vi "loginOrRegister.vi"(8 "error in":errorcluster, 10 "passwd":string, 11 "uname":string) -> (0 "error out":errorcluster, 3 "OK?":bool)   [LabVIEW 2024]
uses:
  user_name.vi
  session.vi
  <vilib>/regexp/Match Regular Expression.xnode
  <vilib>/httpClient/LabVIEWHTTPClient.lvlib
panel:
  # "Login Or Register"
  # "Login or register to server, check internet status,\nafter successfully logged in, save session as global variable, save user name as global variable, download user avatar from server"
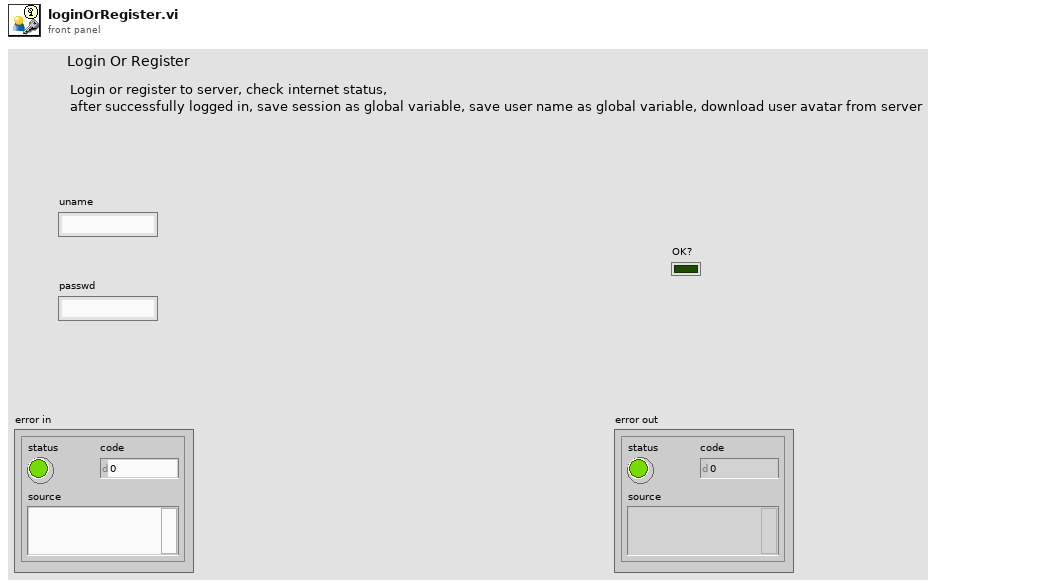
[diagram p1: front panel]
types:
  T1 = typedef "LabVIEWHTTPClient.lvlib/ClientHandle.ctl" = refnum<k1>
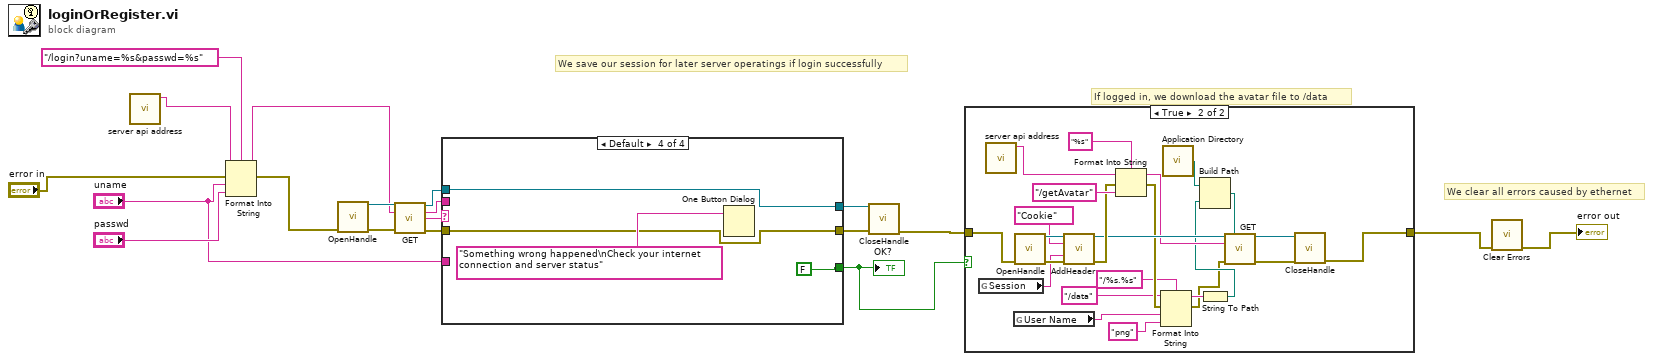
[diagram p0: block diagram]
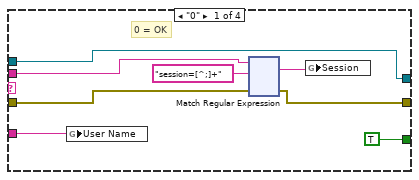
[diagram p2: hidden frame]
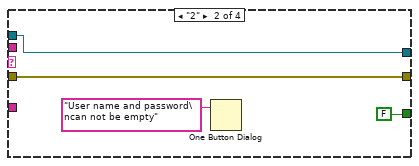
[diagram p3: hidden frame]
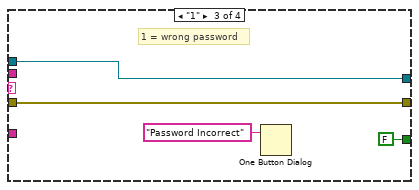
[diagram p4: hidden frame]
diagram:
  # "We clear all errors caused by ethernet"
  # "If logged in, we download the avatar file to /data"
  # "We save our session for later server operatings if login successfully"
  n1 = call "server api address.vi"() -> ("Server API URL"=w4:string)  [unwired: 11 in]
  n2 = Format Into String(format string="/login?uname=%s&passwd=%s", initial string=w4, error in="error in", "uname", "passwd") -> (resulting string=w17:string, error out=w14:errorcluster)
  n3 = call <vilib>:"OpenHandle.vi"("error in (no error)"=w14) -> ("client handle out"=w18:T1, "error out"=w19:errorcluster)  [unwired: 13 in]
  n4 = call <vilib>:"GET.vi"("client handle"=w18, "url"=w17, "error in (no error)"=w19) -> ("client handle out"=w11:T1, "headers"=w12:string, "body"=w13:string, "error out"=w10:errorcluster)  [unwired: 9 in]
  n5 = case shown="Default" w13 {
    tunnel: w12 -> [w24 _ _ _]
    tunnel: w11 -> [w21 w148 w151 w154]
    tunnel: w10 -> [w23 w147 w150 w155]
    tunnel: [TRUE FALSE FALSE FALSE] -> w6
    tunnel: [w21 w148 w151 w154] -> w9
    tunnel: [w22 w147 w150 w155] -> w8
    tunnel: "uname" -> [w20 _ _ _]
    frame "0" {
      # "0 = OK"
      n6 = global write "user_name.vi" "User Name"(w20) -> ()
      n7 = xnode "Match Regular Expression"("input string"=w24, "regular expression"="session=[^;]+", "error in"=w23) -> ("whole match"=w25:string, "error out"=w22:errorcluster)  [unwired: 3 in, 3 out]
      n8 = global write "session.vi" "Session"(w25) -> ()
    }
    frame "2" {
      n9 = One Button Dialog(message="User name and password\ncan not be empty") -> ()  [unwired: 1 in, 1 out]
    }
    frame "1" {
      # "1 = wrong password"
      n10 = One Button Dialog(message="Password Incorrect") -> ()  [unwired: 1 in, 1 out]
    }
    frame Default {
      n11 = One Button Dialog(message="Something wrong happened\nCheck your internet connection and server status") -> ()  [unwired: 1 in, 1 out]
    }
  }
  "OK?" <- w6
  n12 = call <vilib>:"CloseHandle.vi"("client handle"=w9, "error in (no error)"=w8) -> ("error out"=w3:errorcluster)  [unwired: 13 in]
  n13 = case shown="True" w6 {
    tunnel: w3 -> [w157 w181]
    tunnel: [w157 w170] -> w1
    frame False {
    }
    frame True {
      n14 = global read "session.vi" "Session"() -> (w176:string)
      n15 = call "server api address.vi"() -> ("Server API URL"=w158:string)  [unwired: 11 in]
      n16 = global read "user_name.vi" "User Name"() -> (w160:string)
      n17 = call <vilib>:"OpenHandle.vi"("error in (no error)"=w181) -> ("client handle out"=w179:T1, "error out"=w178:errorcluster)  [unwired: 13 in]
      n18 = call <vilib>:"AddHeader.vi"("client handle"=w179, "header"="Cookie", "value"=w176, "error in (no error)"=w178) -> ("client handle out"=w173:T1, "error out"=w174:errorcluster)  [unwired: 10 in]
      n19 = Format Into String(format string="%s", initial string=w158, error in=w174, "/getAvatar" ("input 1")) -> (resulting string=w172:string, error out=w163:errorcluster)
      n20 = Format Into String(format string="/%s.%s", initial string="/data", error in=w163, w160, "png" ("input 2")) -> (resulting string=w165:string, error out=w164:errorcluster)
      n21 = call <vilib>:"Application Directory.vi"() -> ("Application Directory"=w167:path)
      n22 = String To Path(string=w165) -> (path=w166:path)
      n23 = Build Path(base path=w167, name or relative path=w166) -> (appended path=w168:path)
      n24 = call <vilib>:"GET.vi"("client handle"=w173, "output file"=w168, "url"=w172, "error in (no error)"=w164) -> ("client handle out"=w169:T1, "error out"=w171:errorcluster)  [unwired: 8 in, 2 out]
      n25 = call <vilib>:"CloseHandle.vi"("client handle"=w169, "error in (no error)"=w171) -> ("error out"=w170:errorcluster)  [unwired: 13 in]
    }
  }
  n26 = call <vilib>:"Clear Errors.vi"("error in (no error)"=w1) -> ("error out"=→"error out":errorcluster)  [unwired: 5 in, 1 out]
